vi "Read Value (variant).vi"(8 "error in (no error)":errorcluster, 11 "Float D Element in":refnum<class "Float D Element.lvclass">) -> (0 "error out":errorcluster, 2 "Variant":variant, 3 "Float D Element out":refnum<class "Float D Element.lvclass">)   [LabVIEW 2018, in "D Datagrid Library.lvlib" / "Float D Element.lvclass"]
uses:
  Float D Element.lvclass
  Float D Element.lvclass/Float D Element.ctl
  Read Value.vi
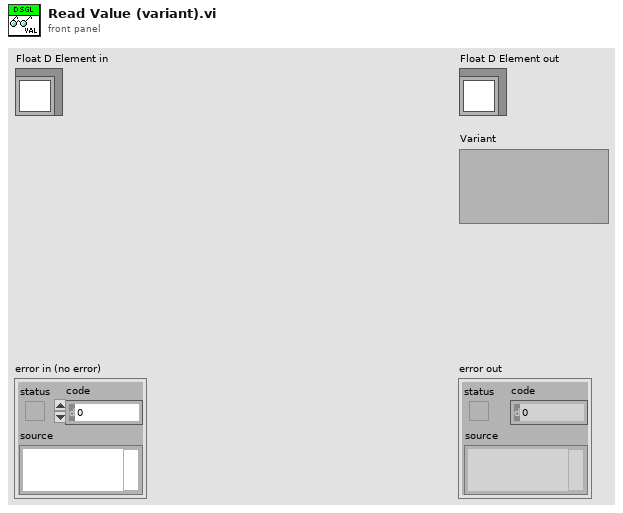
[diagram p1: front panel]
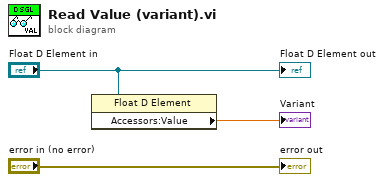
[diagram p0: block diagram]
diagram:
  n1 = property class="Float D Element"(reference="Float D Element in") -> ("Accessors:Value"=→"Variant":sgl)  [unwired: 1 in, 2 out]
  "error out" <- "error in (no error)"
  "Float D Element out" <- "Float D Element in"
